vi "10pt Mov Avg - 2.vi"(10 "Value in":dbl) -> (2 "Value out":dbl)   [LabVIEW 2014]
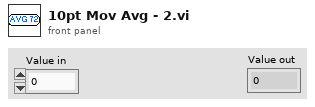
[diagram p1: front panel]
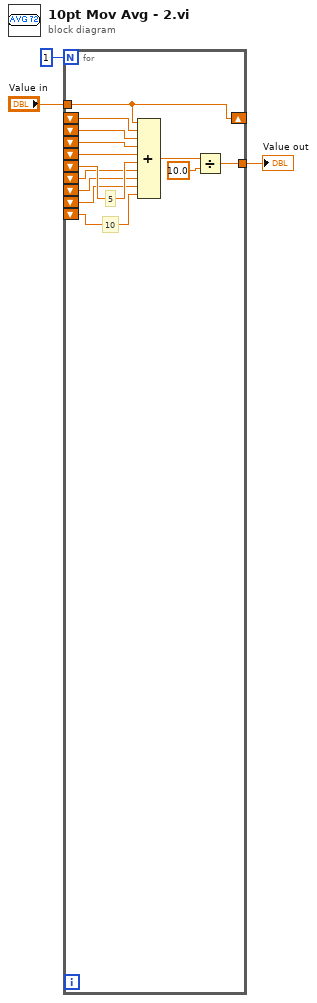
[diagram p0: block diagram]
diagram:
  n1 = for {
    N: 1 -> [_]
    tunnel: "Value in" -> [w16]
    shift-right: [w16] -> _
    shift-left: _ -> [w15]
    shift-left: _ -> [w14]
    shift-left: _ -> [w13]
    shift-left: _ -> [w12]
    tunnel: [w9] -> w1
    shift-left: _ -> [w8]
    shift-left: _ -> [w7]
    shift-left: _ -> [w6]
    shift-left: _ -> [w5]
    shift-left: _ -> [w4]
    # "10"
    # "5"
    n2 = Compound Arithmetic op=ADD(w16, w15, w14, w13, w12, w8, w7, w6, w5, w4) -> (w11:dbl)
    n3 = Divide(x=w11, y=10.0) -> (x/y=w9:dbl)
  }
  "Value out" <- w1
